vi "main_update_env_tree.vi"(10 "Env. Tree":refnum<vi>, 11 "Env_path":path) -> ()   [LabVIEW 2019]
panel:
  # "*******************************************************************\nBiogas Plant Control\n\nAuthor: Paul Zügel\nGCSC-Frankfurt am Main 2020\n\n*******************************************************************"
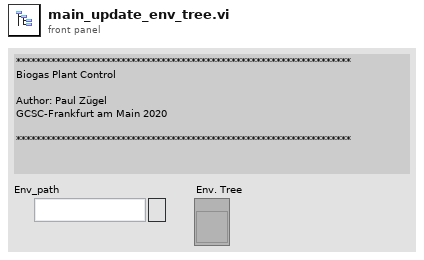
[diagram p1: front panel]
types:
  T1 = cluster{"Left Cell String":string, "Child Text":string[], "Child Tag":string, "Item Indent":i32, "Child Only?":bool, "Glyph Index":i32}
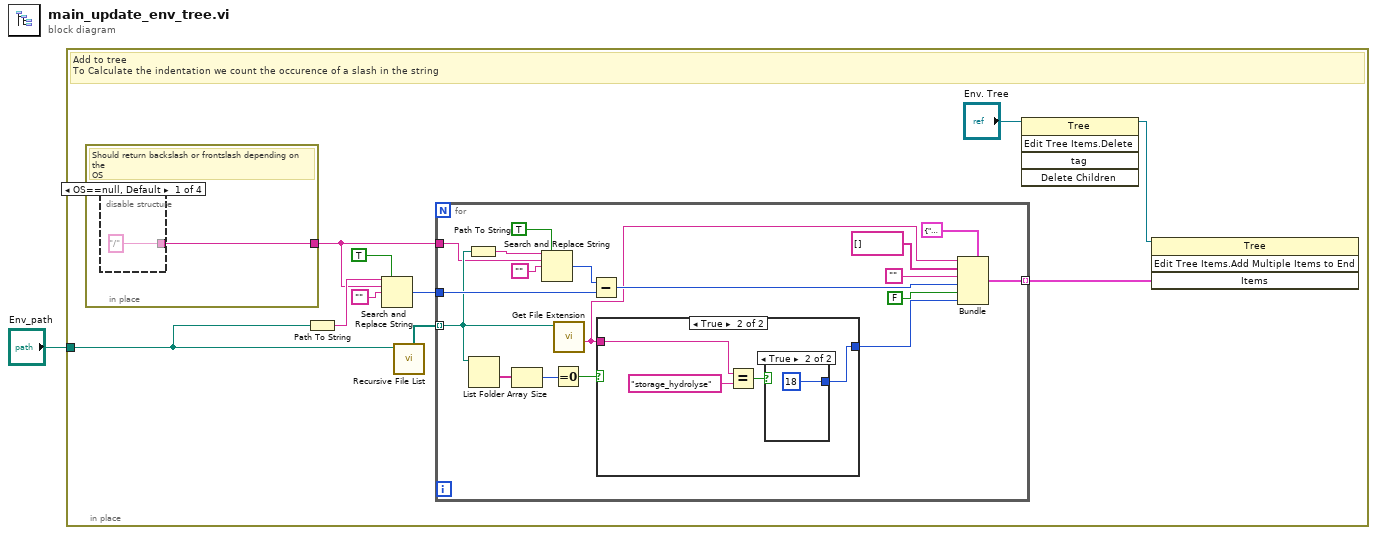
[diagram p0: block diagram]
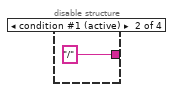
[diagram p2: hidden frame]
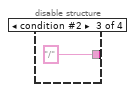
[diagram p3: hidden frame]
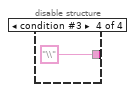
[diagram p4: hidden frame]
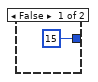
[diagram p5: hidden frame]
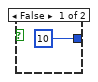
[diagram p6: hidden frame]
diagram:
  n1 = in-place {
    in-place-border: "Env_path" -> [w6]
    # "Add to tree\nTo Calculate the indentation we count the occurence of a slash in the string"
    n2 = in-place {
      in-place-border: [w12] -> w2
      # "Should return backslash or frontslash depending on the\nOS"
      n3 = disable-structure shown="OS==null, Default" {
        disable-tunnel: ["/" ("name or relative path") "/" ("name or relative path") "/" ("name or relative path") "\\" ("name or relative path")] -> w12
        frame condition #0 {
        }
        frame condition #1 (active) {
        }
        frame condition #2 {
        }
        frame condition #3 {
        }
      }
    }
    n4 = Path To String(path=w6) -> (string=w10:string)
    n5 = Search and Replace String(replace all?=TRUE ("replace all? (F)"), input string=w10, search string=w2, replace string="") -> (number of replacements=w7:i32)  [unwired: 4 in, 3 out]
    n6 = call <vilib>:"Recursive File List.vi"("Folder Path"=w6) -> ("All Folders"=w11:path[])  [unwired: 6 in, 4 out]
    n7 = for {
      tunnel: w11 -> [w20] mode=indexing
      tunnel: w7 -> [w30]
      tunnel: [w29] -> w3 mode=indexing
      tunnel: w2 -> [w17]
      n8 = Path To String(path=w20) -> (string=w34:string)
      n9 = List Folder(path=w20) -> (folder names=w19:string[])  [unwired: 3 in, 3 out]
      n10 = Array Size(array=w19) -> (size(s)=w23:i32)
      n11 = Search and Replace String(replace all?=TRUE ("replace all? (F)"), input string=w34, search string=w17, replace string="") -> (number of replacements=w31:i32)  [unwired: 4 in, 3 out]
      n12 = Equal To 0?(x=w23) -> (x = 0?=w22:bool)
      n13 = call <vilib>:"Get File Extension.vi"("file"=w20) -> ("filename without extension"=w18:string)  [unwired: 6 in, 4 out]
      n14 = Subtract(x=w31, y=w30) -> (x-y=w28:i32)
      n15 = case shown="True" w22 {
        tunnel: [15 ("Glyph Index") w36] -> w21
        tunnel: w18 -> [_ w39]
        frame False {
        }
        frame True {
          n16 = Equal?(x=w39, y="storage_hydrolyse") -> (x = y?=w37:bool)
          n17 = case shown="True" w37 {
            tunnel: [10 ("Glyph Index") 18 ("Glyph Index")] -> w36
            frame False {
            }
            frame True {
            }
          }
        }
      }
      n18 = Bundle(cluster=T1 {"Left Cell String"="", "Child Text"=[], "Child Tag"="", "Item Indent"=0, "Child Only?"=FALSE, "Glyph Index"=0} ("Item"), "Left Cell String"=w18, "Child Text"=string[] [], "Child Tag"="", "Item Indent"=w28, "Child Only?"=FALSE, "Glyph Index"=w21) -> (w29:T1)
    }
    n19 = invoke class="Tree" method="Edit Tree Items.Delete"(reference="Env. Tree") -> (reference out=w4:refnum<vi>)  [unwired: 4 in, 4 out]
    n20 = invoke class="Tree" method="Edit Tree Items.Add Multiple Items to End"(reference=w4, "Items"=w3) -> ()  [unwired: 2 in, 4 out]
  }
